vi "even odd check.vi"(11 "position":dbl) -> (3 "index":i32)   [LabVIEW 2021]
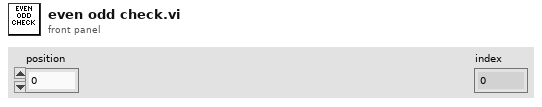
[diagram p1: front panel]
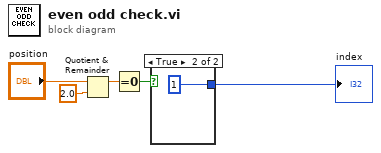
[diagram p0: block diagram]
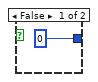
[diagram p2: hidden frame]
diagram:
  n1 = Quotient & Remainder(x="position", y=2.0) -> (x-y*floor(x/y)=w4:dbl)  [unwired: 1 out]
  n2 = Equal To 0?(x=w4) -> (x = 0?=w5:bool)
  n3 = case shown="True" w5 {
    tunnel: [0 1] -> w1
    frame False {
    }
    frame True {
    }
  }
  "index" <- w1
